vi "XYsave.vi"(2 "error in":errorcluster, 3 "Cluster":T1, 4 "datalog path (use dialog)":path) -> (0 "error out":errorcluster, 1 "offset (in records)":i64)   [LabVIEW 2013]
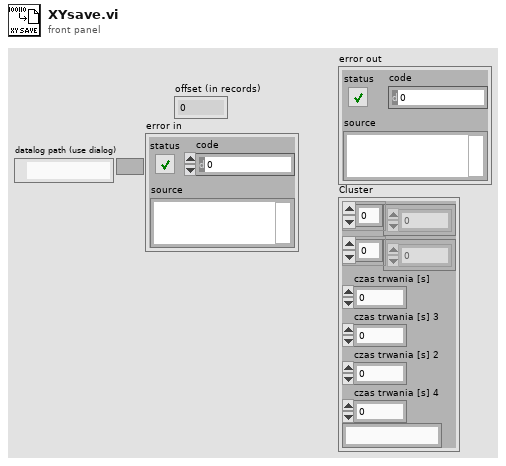
[diagram p1: front panel]
types:
  T1 = cluster{dbl[], dbl[], "czas trwania [s]":dbl, "czas trwania [s] 3":dbl, "czas trwania [s] 2":dbl, "czas trwania [s] 4":dbl, string}
  T2 = enum16{"open", "replace", "create", "open or create", "replace or create", "replace or create with confirmation"}
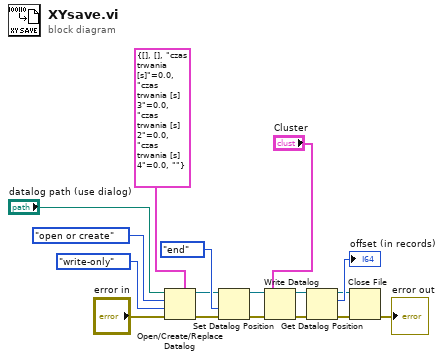
[diagram p0: block diagram]
diagram:
  n1 = Open/Create/Replace Datalog(5:T1 {[], [], "czas trwania [s]"=0.0, "czas trwania [s] 3"=0.0, "czas trwania [s] 2"=0.0, "czas trwania [s] 4"=0.0, ""} ("Cluster"), 8:"error in", 9:enum16{"read/write", "read-only", "write-only"}."write-only" ("access (0:read/write)"), 10:T2."open or create" ("operation (0:open)"), 11:"datalog path (use dialog)") -> (0:w9:errorcluster, 3:w7:refnum<k1>)  [unwired: 1 in, 1 out]
  n2 = Set Datalog Position(4:w9, 5:enum16{"start", "end", "current"}."end" ("from (0:start)"), 7:w7) -> (0:w17:errorcluster, 3:w8:refnum<k1>)  [unwired: 1 in]
  n3 = Write Datalog(4:w17, 6:"Cluster", 7:w8) -> (0:w12:errorcluster, 3:w11:refnum<k1>)
  n4 = Get Datalog Position(4:w12, 7:w11) -> (0:w14:errorcluster, 2:→"offset (in records)":i64, 3:w13:refnum<k1>)
  n5 = Close File(refnum=w13, error in=w14) -> (error out=→"error out":errorcluster)  [unwired: 1 out]
